vi "Stop.vi"(1 "stop":bool) -> (0 "Fim":bool)   [LabVIEW 2018]
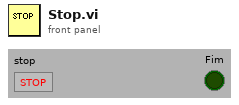
[diagram p1: front panel]
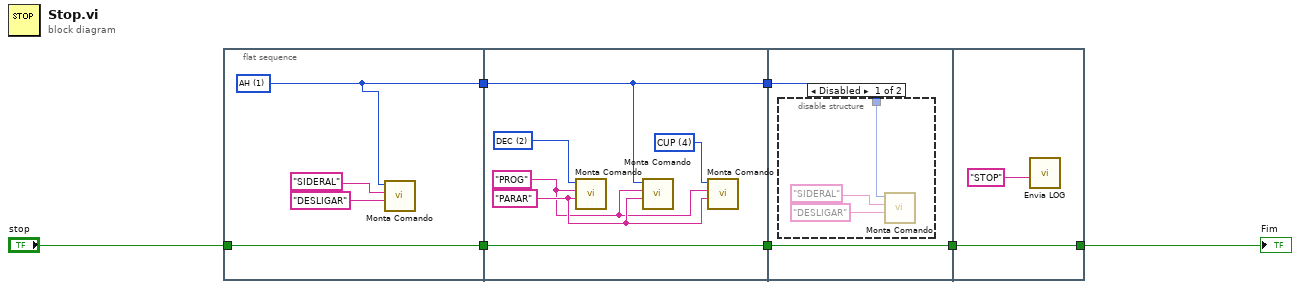
[diagram p0: block diagram]
diagram:
  n1 = flat-sequence {
    tunnel: "stop" -> [w11]
    tunnel: [w11] -> w3
    tunnel: [w8] -> w2
    tunnel: [w12] -> w7
    tunnel: [w13] -> w5
    tunnel: w3 -> [w13]
    tunnel: w2 -> [w12]
    tunnel: w7 -> [w19]
    tunnel: [w18] -> w1
    tunnel: w5 -> [w18]
    tunnel: w1 -> [w23]
    tunnel: [w23] -> w4
    frame #0 {
      w8 = u16 1 items=["ZERO", "AH", "DEC", "TUBO", "CUP"] ("Controlador")
      n2 = call "Monta Comando.vi"("Comando"="DESLIGAR", "Dispositivo"="SIDERAL" ("Set Point"), "Controlador"=w8) -> ()  [unwired: 2 in, 5 out]
    }
    frame #1 {
      w15 = u16 4 items=["ZERO", "AH", "DEC", "TUBO", "CUP"] ("Controlador")
      w17 = "PARAR" ("Comando")
      w14 = u16 2 items=["ZERO", "AH", "DEC", "TUBO", "CUP"] ("Controlador")
      w16 = "PROG" ("Dispositivo")
      n3 = call "Monta Comando.vi"("Comando"=w17, "Dispositivo"=w16, "Controlador"=w14) -> ()  [unwired: 2 in, 5 out]
      n4 = call "Monta Comando.vi"("Comando"=w17, "Dispositivo"=w16, "Controlador"=w12) -> ()  [unwired: 2 in, 5 out]
      n5 = call "Monta Comando.vi"("Comando"=w17, "Dispositivo"=w16, "Controlador"=w15) -> ()  [unwired: 2 in, 5 out]
    }
    frame #2 {
      n6 = disable-structure shown="Disabled" {
        disable-tunnel: w19 -> [w20 _]
        frame Disabled {
          n7 = call "Monta Comando.vi"("Comando"="DESLIGAR", "Dispositivo"="SIDERAL" ("Set Point"), "Controlador"=w20) -> ()  [unwired: 2 in, 5 out]
        }
        frame Enabled {
        }
      }
    }
    frame #3 {
      n8 = call "Envia LOG.vi"("Comando a ser logado"="STOP" ("string")) -> ()  [unwired: 7 in, 2 out]
    }
  }
  "Fim" <- w4
